vi "All Child Values.vi"(11 "NewEntityTemplate in":refnum<class "NewEntityTemplate.lvclass">) -> (2 "All Values":refnum<class "Type.lvclass">[](array[class]))   [LabVIEW 2020, in "Conditum-Tools.lvlib" / "NewEntityTemplate.lvclass"]
uses:
  NewEntityTemplate.lvclass
  Conditum/Columns/Type/Type.lvclass
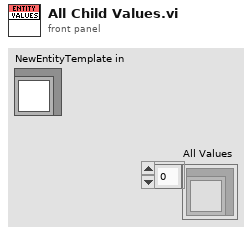
[diagram p1: front panel]
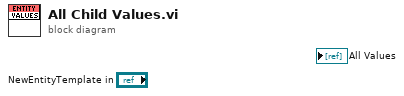
[diagram p0: block diagram]
diagram:
